vi "test_AK TCP Protocol Factory.vi"(8 "error in (no error)":errorcluster, 11 "TestCase in":refnum<class "Instrument Addon Scripting API Protocol Factories Unit Tests.lvclass">) -> (0 "error out":errorcluster, 3 "TestCase out":refnum<class "Instrument Addon Scripting API Protocol Factories Unit Tests.lvclass">)   [LabVIEW 2018, in "Instrument Addon Scripting API Protocol Factories Unit Tests.lvclass"]
uses:
  Instrument Addon Scripting API Protocol Factories Unit Tests.lvclass
  AK TCP/AK TCP Settings.ctl
  AK TCP/AK TCP.lvclass
  D:/GitRepository/niveristand-instrument-addon-classes/Source/Protocols/TCP/TCP.lvclass
  TCP/TCP.lvclass/TCP.ctl
  TCP/Data Access/Read IP Address.vi
  TCP/Data Access/Read Port.vi
  <vilib>/addons/_JKI Toolkits/VI Tester/TestCase.llb/TestCase.lvclass
  C:/Program Files (x86)/National Instruments/LabVIEW 2018/vi.lib/addons/_JKI Toolkits/VI Tester/TestCase.llb/TestCase.lvclass
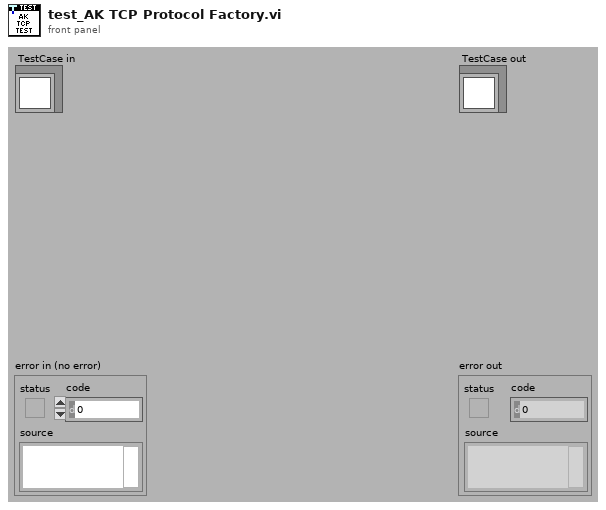
[diagram p1: front panel]
types:
  T1 = typedef "Protocols.lvlib/AK TCP.lvclass/AK TCP Settings.ctl" = cluster{"IP Address":string, "Port":u16}
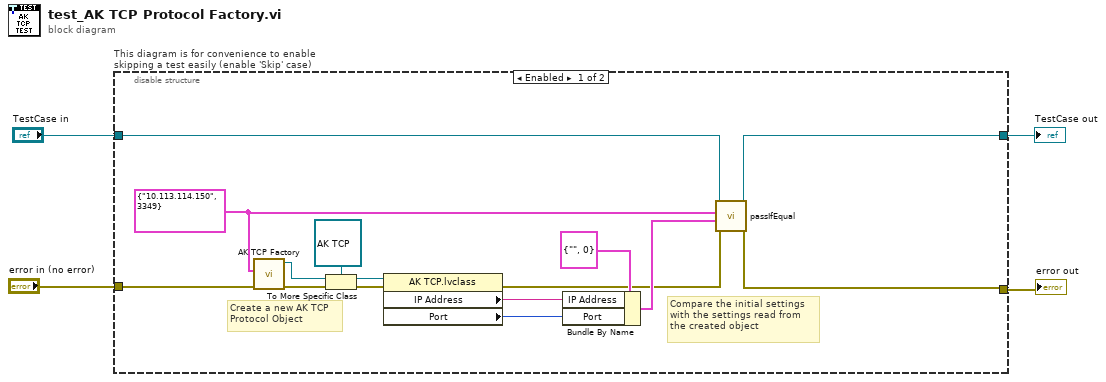
[diagram p0: block diagram]
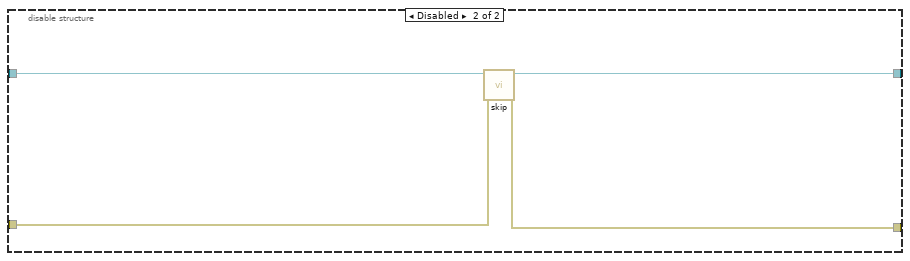
[diagram p2: hidden frame]
diagram:
  n1 = disable-structure "This diagram is for convenience to enable skipping a test easily (enable 'Skip' case)" shown="Enabled" {
    disable-tunnel: "TestCase in" -> [w19 w23]
    disable-tunnel: [w18 w21] -> w1
    disable-tunnel: [w17 w22] -> w3
    disable-tunnel: "error in (no error)" -> [w16 w20]
    frame Enabled {
      w13 = T1 {"IP Address"="10.113.114.150", "Port"=3349} ("AK TCP Settings")
      # "Compare the initial settings \nwith the settings read from \nthe created object"
      # "Create a new AK TCP\nProtocol Object"
      n2 = call "AK TCP Factory.vi"("error in (no error)"=w16, "AK TCP settings"=w13) -> ("error out"=w7:errorcluster, "protocol out"=w6:refnum<class "Protocol Parent.lvclass">)  [unwired: 8 in]
      n3 = To More Specific Class(target class=refnum<class "AK TCP.lvclass"> refnum ("Protocols.lvlib:AK TCP.lvclass"), reference=w6, error in=w7) -> (specific class reference=w9:refnum<class "AK TCP.lvclass">, error out=w8:errorcluster)
      n4 = property class="AK TCP.lvclass"(reference=w9, error in=w8) -> (error out=w12:errorcluster, "IP Address"=w11:string, "Port"=w10:u16)  [unwired: 1 out]
      n5 = Bundle By Name(cluster=T1 {"IP Address"="", "Port"=0} ("AK TCP Settings"), "IP Address"=w11, "Port"=w10) -> (w14:T1)
      n6 = call-dynamic "passIfEqual.vi"("error in (no error)"=w12, "y"=w14, "x"=w13, "TestCase in"=w19) -> ("error out"=w17:errorcluster, "TestCase out"=w18:refnum<class "Instrument Addon Scripting API Protocol Factories Unit Tests.lvclass">)  [unwired: 6 in]
    }
    frame Disabled {
      # "skip test result while test is under development"
      n7 = call <vilib>:"skip.vi"("error in (no error)"=w20, "TestCase in"=w23) -> ("error out"=w22:errorcluster, "TestCase out"=w21:refnum<class "Instrument Addon Scripting API Protocol Factories Unit Tests.lvclass">)  [unwired: 8 in]
    }
  }
  "error out" <- w3
  "TestCase out" <- w1
